vi "Creat XLS by Station.vi"(2 "staiton":T2, 3 "data in":string[](array[string]), 4 "2D data":string[][](array[string]) caption="二维数据") -> (6 "new file path (Not A Path if cancelled)":path caption="新建文件路径（取消时为非法路径）")   [LabVIEW 2018]
uses:
  DefCtrl/Station.ctl
  DefCtrl/ListInf.ctl
panel:
  in  "List Inf":T1={"粗切工位"=["结束时间", "料车号", "切割文件", "项目类型", "过程条码", "来料条码"], "热处理工位"=["生产时间", "料车号", "加热开始时间", "加热结束时间", "设定加热时长", "实际加热时长", "设定加热温度", "项目类型", "过程代码"], "精切工位"=["结束时间", "上料料盘号A", "料盘A开始时间", "上料料盘号B", "料盘B开始时间", "切割文件", "项目类型", "下料料车号", "过程代码"], "PDF工位"={"List 1"=["生产时间", "料车号", "项目类型", "过程条码", "焊接开始时间", "焊接结束时间"], "List 2"=["压型进口温度1", "压型进口温度2", "压型进口温度3", "压型进口温度4", "压型进口温度5", "压型进口温度6", "压型进口温度7", "压型进口温度8", "压型进口温度9", "压型进口温度10", "压型进口温度11", "压型进口温度12", "压型进口温度13", "压型进口温度14", "压型进口温度15", "压型进口温度16", "压型进口温度17", "压型进口温度18", "压型进口温度19", "压型进口温度20", "压型进口温度21", "压型进口温度22", "压型进口温度23", "压型进口温度24", "压型进口温度25", "压型进口温度26", "压型进口温度27", "压型进口温度28", "压型进口温度29", "压型进口温度30"], "List 3"=["焊接出口温度1", "焊接出口温度2", "焊接出口温度3", "焊接出口温度4", "焊接出口温度5", "焊接出口温度6", "焊接出口温度7", "焊接出口温度8", "焊接出口温度9", "焊接出口温度10", "焊接出口温度11", "焊接出口温度12", "焊接出口温度13", "焊接出口温度14", "焊接出口温度15", "焊接出口温度16", "焊接出口温度17", "焊接出口温度18", "焊接出口温度19", "焊接出口温度20", "焊接出口温度21", "焊接出口温度22", "焊接出口温度23", "焊接出口温度24", "焊接出口温度25", "焊接出口温度26", "焊接出口温度27", "焊接出口温度28", "焊接出口温度29", "焊接出口温度30"], "List 4"=["压力值1", "压力值2", "压力值3", "压力值4", "压力值5", "压力值6", "压力值7", "压力值8", "压力值9", "压力值10", "压力值11", "压力值12", "压力值13", "压力值14", "压力值15", "压力值16", "压力值17", "压力值18", "压力值19", "压力值20", "压力值21", "压力值22", "压力值23", "压力值24", "压力值25", "压力值26", "压力值27", "压力值28", "压力值29", "压力值30"]}, "打凹点工位"=["生产时间", "扭矩值", "圈数", "当前项目"], "检测工位"=["流水号", "时间", "收回1力值", "收回2力值", "收回3力值", "收回4力值", "展开1力值", "展开2力值", "展开3力值", "展开4力值", "项目号", "Pass/Fail"]}
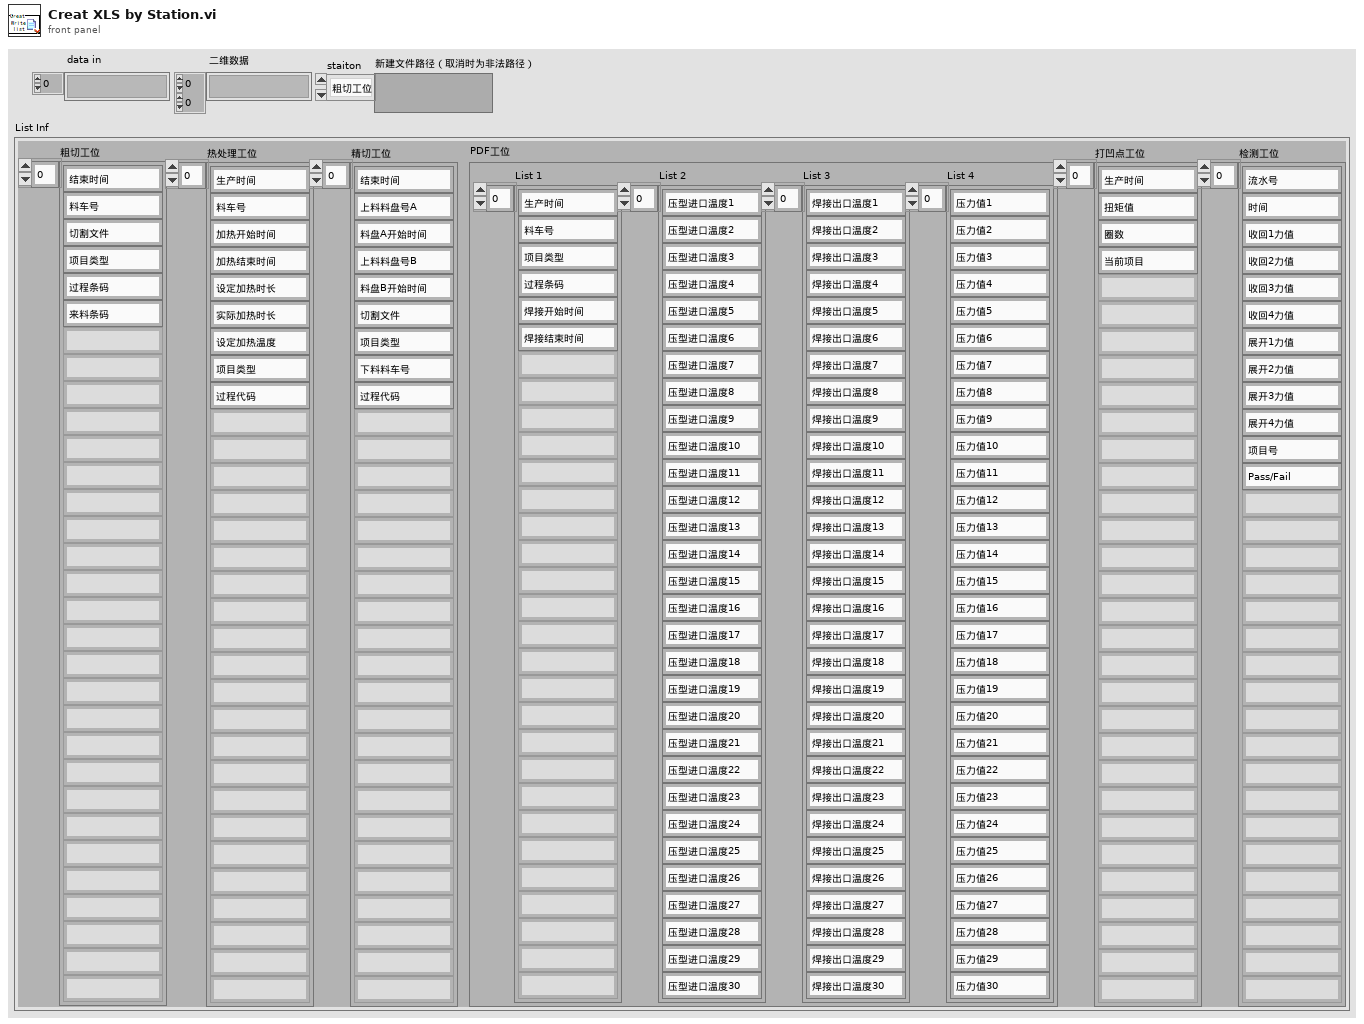
[diagram p1: front panel]
types:
  T1 = typedef "ListInf.ctl" = cluster{"粗切工位":string[], "热处理工位":string[], "精切工位":string[], "PDF工位":cluster{"List 1":string[], "List 2":string[], "List 3":string[], "List 4":string[]}, "打凹点工位":string[], "检测工位":string[]}
  T2 = typedef "Station.ctl" = enum16{"粗切工位", "热处理工位", "精切工位", "PDF焊接工位", "打凹点预载力工位", "收卷工位", "EOL工位"}
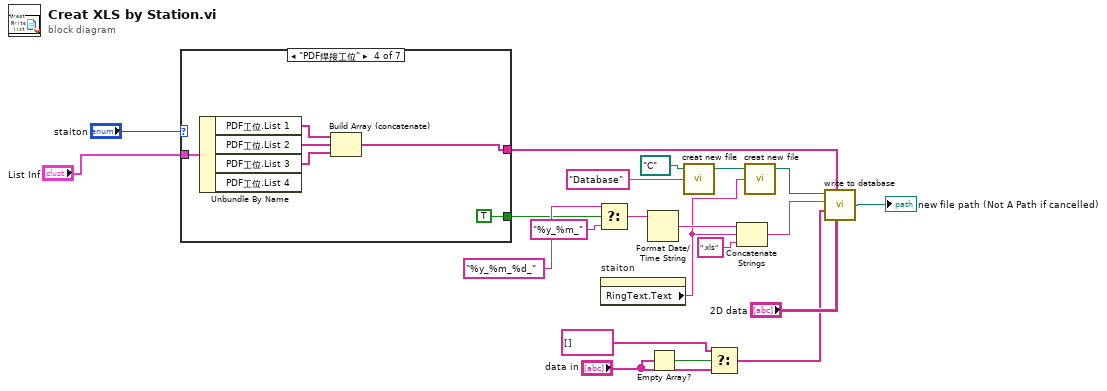
[diagram p0: block diagram]
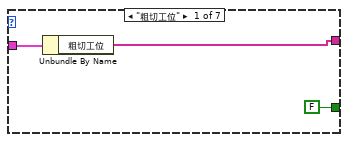
[diagram p2: hidden frame]
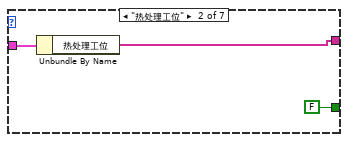
[diagram p3: hidden frame]
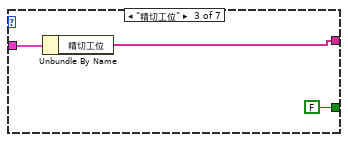
[diagram p4: hidden frame]
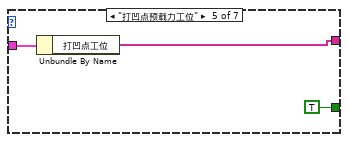
[diagram p5: hidden frame]
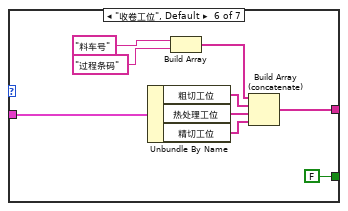
[diagram p6: hidden frame]
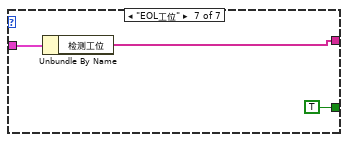
[diagram p7: hidden frame]
diagram:
  n1 = case shown="\"PDF焊接工位\"" "staiton" {
    tunnel: [w23 w26 w29 w32 w38 w48 w50] -> w9
    tunnel: [FALSE FALSE FALSE TRUE TRUE FALSE TRUE] -> w7
    tunnel: "List Inf" -> [w22 w25 w28 w31 w37 w40 w49]
    frame "粗切工位" {
      n2 = Unbundle By Name(w22) -> ("粗切工位"=w23:string[])
    }
    frame "热处理工位" {
      n3 = Unbundle By Name(w25) -> ("热处理工位"=w26:string[])
    }
    frame "精切工位" {
      n4 = Unbundle By Name(w28) -> ("精切工位"=w29:string[])
    }
    frame "PDF焊接工位" {
      n5 = Unbundle By Name(w31) -> ("PDF工位.List 1"=w35:string[], "PDF工位.List 2"=w34:string[], "PDF工位.List 3"=w33:string[])  [unwired: 1 out]
      n6 = Build Array (concatenate)(w35, w34, w33) -> (w32:string[])
    }
    frame "打凹点预载力工位" {
      n7 = Unbundle By Name(w37) -> ("打凹点工位"=w38:string[])
    }
    frame "收卷工位", Default {
      n8 = Unbundle By Name(w40) -> ("粗切工位"=w46:string[], "热处理工位"=w45:string[], "精切工位"=w44:string[])
      n9 = Build Array("料车号", "过程条码") -> (w41:string[])
      n10 = Build Array (concatenate)(w41, w46, w45, w44) -> (w48:string[])
    }
    frame "EOL工位" {
      n11 = Unbundle By Name(w49) -> ("检测工位"=w50:string[])
    }
  }
  n12 = Select(t="%y_%m_%d_" ("时间格式字符串(%c)"), s=w7, f="%y_%m_" ("时间格式字符串(%c)")) -> (s? t:f=w14:string)
  n13 = property on="staiton" class="Enum (严格)"() -> ("RingText.Text"=w6:string)  [unwired: 2 in, 2 out]
  n14 = Format Date/Time String(time format string (%c)=w14) -> (date/time string=w19:string)  [unwired: 2 in]
  n15 = Empty Array?(array="data in") -> (empty?=w4:bool)
  n16 = call "creat new file.vi"("file name"="Database", "path"=path "C:/") -> ("created path"=w16:path)  [unwired: 1 in, 2 out]
  n17 = Select(t=string[] [], s=w4, f="data in") -> (s? t:f=w2:string[])
  n18 = Concatenate Strings(w19, w6, ".xls" ("字符串")) -> (w17:string)
  n19 = call "creat new file.vi"("file name"=w6, "path"=w16) -> ("created path"=w15:path)  [unwired: 1 in, 2 out]
  n20 = call "write to database.vi"("2D data"="2D data", "Header"=w9, "data in"=w2, "file name"=w17, "path"=w15) -> ("new file path (Not A Path if cancelled)"=→"new file path (Not A Path if cancelled)":path)  [unwired: 1 in]
